vi "Get Category.vi"(8 "error in (no error)":errorcluster, 11 "Daqmx Module editor node in":refnum<class "DAQmx Module Editor Node.lvclass">) -> (0 "error out":errorcluster, 2 "Category":string, 3 "Daqmx Module editor node out":refnum<class "DAQmx Module Editor Node.lvclass">)   [LabVIEW 2014, in "DAQmx Module Editor Node.lvclass"]
uses:
  DAQmx Module Editor Node.lvclass
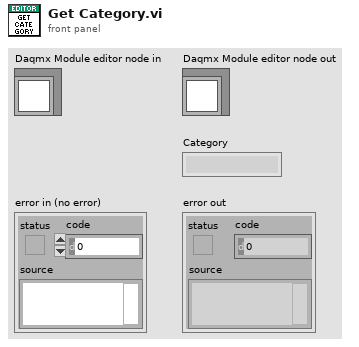
[diagram p1: front panel]
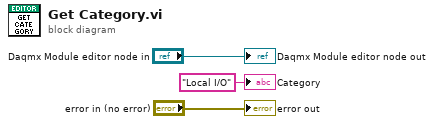
[diagram p0: block diagram]
diagram:
  "error out" <- "error in (no error)"
  "Daqmx Module editor node out" <- "Daqmx Module editor node in"
  "Category" <- "Local I/O" ("Category")
